vi "TestRun HovaCAL SystemValues.vi"() -> (3 "Info Cluster":T1)   [LabVIEW 2020, in "Linearisierung v2.lvlib" / "Gasteiler.lvlib" / "HovaCAL_Interface.lvlib"]
uses:
  HovaCAL_Interface.lvlib
  Controls/Info Cluster.ctl
  Controls/Controls.lvlib
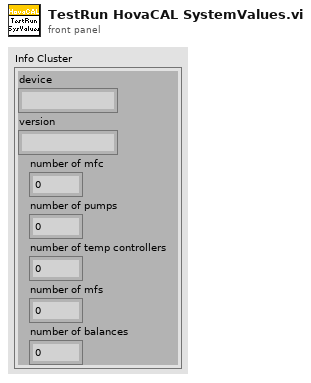
[diagram p1: front panel]
types:
  T1 = typedef "Linearisierung v2.lvlib/Gasteiler.lvlib/HovaCAL_Interface.lvlib/Controls.lvlib/Info Cluster.ctl" = cluster{"device":string, "version":string, "number of mfc":i32, "number of pumps":i32, "number of temp controllers":i32, "number of mfs":i32, "number of balances":i32}
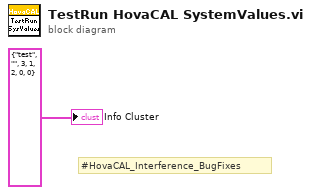
[diagram p0: block diagram]
diagram:
  # "#HovaCAL_Interference_BugFixes"
  "Info Cluster" <- T1 {"device"="test", "version"="", "number of mfc"=3, "number of pumps"=1, "number of temp controllers"=2, "number of mfs"=0, "number of balances"=0} ("Info Cluster")
